vi "Loop_SEN.vi"() -> ()   [LabVIEW 2017, in "Dashboard.lvlib"]
uses:
  Dashboard.lvlib
  Globals/Global_STOP.vi
  Compressor/Globals/GLOBAL_ACT Write_Data_Out.vi
  Globals/Global_CMD_Drive.vi
  System_Monitoring/Global_SEN Write_Data.vi
  Globals/Global_CMD_Gear.vi
  Compressor/Compressor.lvlib
  System_Monitoring/System_Status.lvlib
panel:
  out "Cycle Time (S)":dbl format="%.3g"
  in  "Target Time(ms)":u32=50
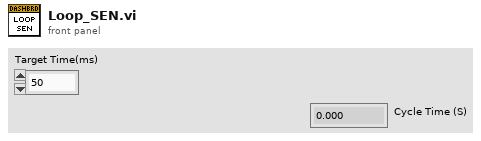
[diagram p1: front panel]
types:
  T1 = cluster{"Target Time(ms)":u32, "Current Time":timestamp, "Previous Time":timestamp, "Cycle Time (S)":dbl, "Num NET Vars":i32}
  T2 = typedef "Cluster_Compressor.ctl" = cluster{"Compressor Running":bool, "Compressor Enabled":bool}
  T3 = typedef "CLUSTER_CMD_WC_Drive.ctl" = cluster{"Drive_Mode":T4, "VBus":T5, "Profile":T7}
  T4 = typedef "ENUM_WC_Drive_DriveMode.ctl" = enum16{"Motion Profile", "CrossLineAuto", "VBus", "Stop"}
  T5 = typedef "CLUSTER_Drive_ACT Loop_VBus Data.ctl" = cluster{"Drive":T6, "Turbo":bool}
  T6 = typedef "CLUSTER_X and Y.ctl" = cluster{"Steer":dbl, "Throtle":dbl}
  T7 = typedef "CLUSTER_Drive_ACT Loop_Profile Data.ctl" = cluster{"Start":bool}
  T8 = typedef "CLUSTER_RoboRio_Status.ctl" = cluster{"RoboRio Faults":T9, "RIO inpt vol (V)":dbl, "RIO inpt cur (A)":dbl, "RoboRio Rails":T10}
  T9 = typedef "CLUSTER_RoboRio_Faults.ctl" = cluster{"Inpt. V. Brn. Out":bool, "3.3V Usr Rail Shrt.":bool, "5 V Usr Rail Shrt.":bool, "6 V Usr. Rail Shrt.":bool, "5V Usr. Rail Brn. Out":bool}
  T10 = typedef "CLUSTER_RoboRio_Rails.ctl" = cluster{"3.3 Volt":T11, "5 Volt":T11, "6 Volt":T11}
  T11 = typedef "CLUSTER_RoboRio_SingleRail.ctl" = cluster{"Vol.  (V)":dbl, "Cur. (A)":dbl}
  T12 = typedef "CLUSTER_PCM_Status.ctl" = cluster{"Current (A)":dbl, "All Solenoid Faults":bool[], "Input Voltage":dbl, "Solenoid Voltage":dbl, "Comp. Fault":bool}
  T13 = typedef "CLUSTER_PDP_Status.ctl" = cluster{"PDP Faults":T14, "All Currents (A)":dbl[], "Energy (J)":dbl, "Power (W)":dbl, "Voltage (V)":dbl}
  T14 = typedef "CLUSTER_PDP_Faults.ctl" = cluster{"Current Faults":bool[], "Batt V Fault":bool, "Temp Fault":bool, "HW Fault":bool}
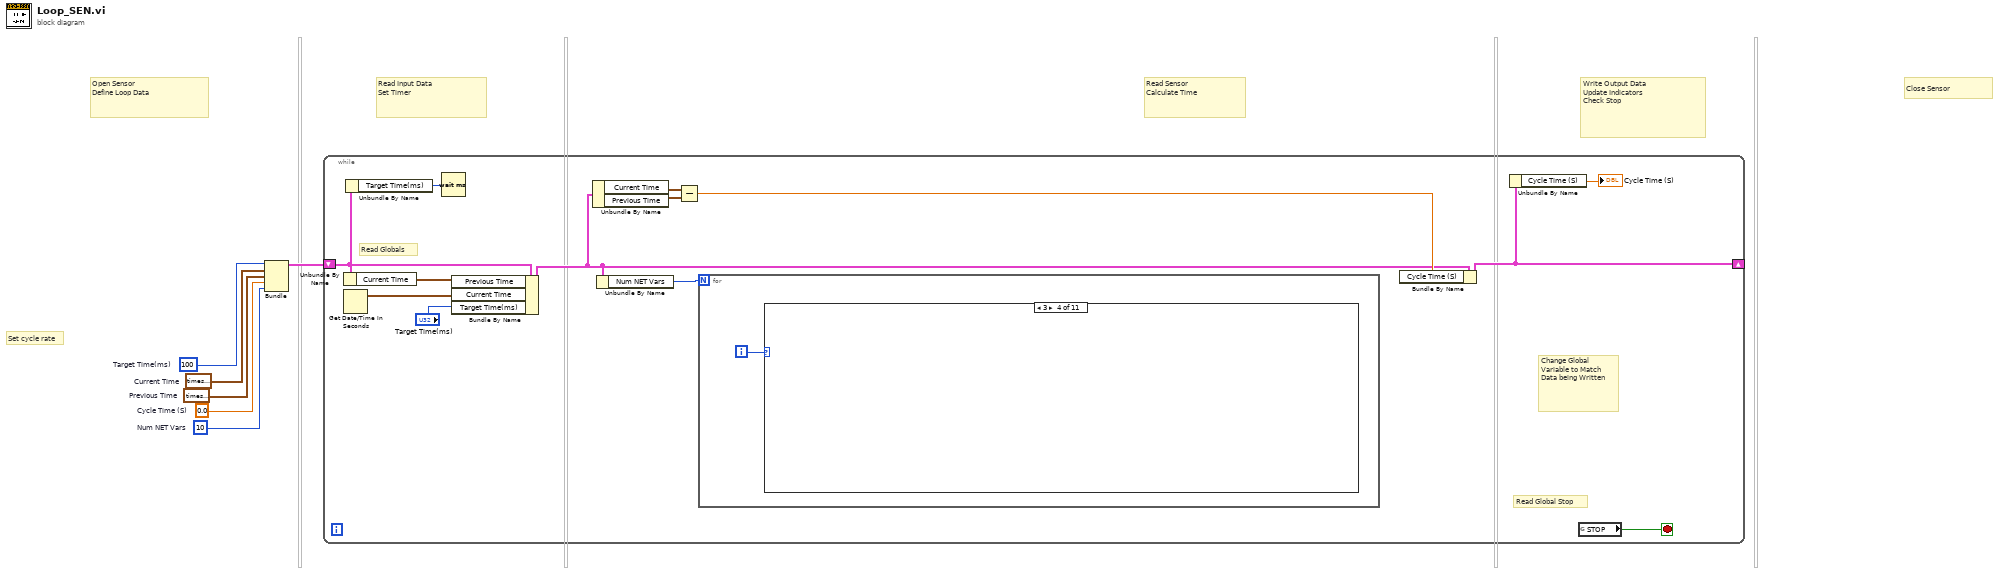
[diagram p0: block diagram]
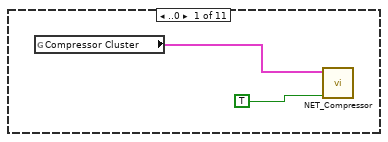
[diagram p2: hidden frame]
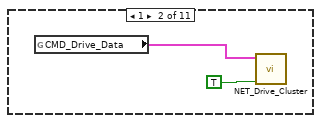
[diagram p3: hidden frame]
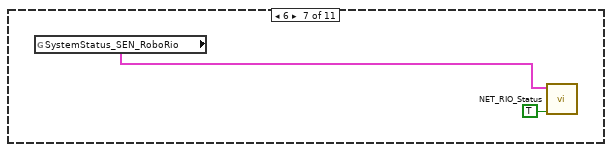
[diagram p7: hidden frame]
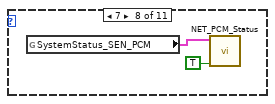
[diagram p8: hidden frame]
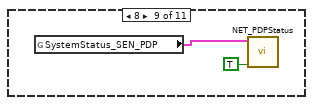
[diagram p9: hidden frame]
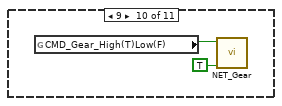
[diagram p10: hidden frame]
diagram:
  w1 = 10  # Num NET Vars
  w2 = 0.0  # Cycle Time (S)
  w6 = timestamp(0 s since 1904-01-01)  # Previous Time
  w5 = timestamp(0 s since 1904-01-01)  # Current Time
  w4 = u32 100  # Target Time(ms)
  # "Close Sensor"
  # "Write Output Data\nUpdate Indicators\nCheck Stop"
  # "Read Sensor\nCalculate Time"
  # "Read Input Data\nSet Timer"
  # "Open Sensor\nDefine Loop Data"
  # "Set cycle rate"
  n1 = Bundle("Target Time(ms)"=w4, "Current Time"=w5, "Previous Time"=w6, "Cycle Time (S)"=w2, "Num NET Vars"=w1) -> (w3:T1)  [unwired: 1 in]
  n2 = while {
    shift-right: [w11] -> _
    shift-left: w3 -> [w13]
    stop <- w19 stop-if-true
    # "Change Global\nVariable to Match\nData being Written"
    # "Read Globals"
    # "Read Global Stop"
    n3 = Unbundle By Name(w13) -> ("Current Time"=w17:timestamp)
    n4 = Get Date/Time In Seconds() -> (seconds since 1Jan1904=w18:timestamp)
    n5 = Unbundle By Name(w13) -> ("Target Time(ms)"=w12:u32)
    n6 = Wait (ms)(milliseconds to wait=w12) -> ()  [unwired: 1 out]
    n7 = Bundle By Name(cluster=w13, "Previous Time"=w17, "Current Time"=w18, "Target Time(ms)"="Target Time(ms)") -> (w8:T1)
    n8 = Unbundle By Name(w8) -> ("Current Time"=w16:timestamp, "Previous Time"=w15:timestamp)
    n9 = Unbundle By Name(w8) -> ("Num NET Vars"=w7:i32)
    n10 = Subtract(x=w16, y=w15) -> (x-y=w9:dbl)
    n11 = for {
      N: w7 -> [_]
      i -> [w20]
      n12 = case shown="3" w20 {
        frame ..0 {
          n13 = global read "GLOBAL_ACT Write_Data_Out.vi" "Compressor Cluster"() -> (w21:T2)
          n14 = call "NET_Compressor.vi"("Read(F) Write(T)"=TRUE, "Compressor  In"=w21) -> ()  [unwired: 9 in, 1 out]
        }
        frame 1 {
          n15 = global read "Global_CMD_Drive.vi" "CMD_Drive_Data"() -> (w23:T3)
          n16 = call "NET_Drive_Cluster.vi"("Read(F) Write(T)"=TRUE, "CMD_DriveCluster"=w23) -> ()  [unwired: 9 in, 1 out]
        }
        frame 2 {
        }
        frame 3 {
        }
        frame 4 {
        }
        frame 5 {
        }
        frame 6 {
          n17 = global read "Global_SEN Write_Data.vi" "SystemStatus_SEN_RoboRio"() -> (w25:T8)
          n18 = call "NET_RIO_Status.vi"("Read(F) Write(T)"=TRUE, "RoboRio Status In"=w25) -> ()  [unwired: 9 in, 1 out]
        }
        frame 7 {
          n19 = global read "Global_SEN Write_Data.vi" "SystemStatus_SEN_PCM"() -> (w28:T12)
          n20 = call "NET_PCM_Status.vi"("Read(F) Write(T)"=TRUE, "PCM_Status_In"=w28) -> ()  [unwired: 9 in, 1 out]
        }
        frame 8 {
          n21 = global read "Global_SEN Write_Data.vi" "SystemStatus_SEN_PDP"() -> (w30:T13)
          n22 = call "NET_PDPStatus.vi"("Read(F) Write(T)"=TRUE, "PDP_Status_In"=w30) -> ()  [unwired: 9 in, 1 out]
        }
        frame 9 {
          n23 = global read "Global_CMD_Gear.vi" "CMD_Gear_High(T)Low(F)"() -> (w31:bool)
          n24 = call "NET_Gear.vi"("Read(F) Write(T)"=TRUE, "High Gear In"=w31) -> ()  [unwired: 9 in, 1 out]
        }
        frame 10.. {
        }
      }
    }
    n25 = Bundle By Name(cluster=w8, "Cycle Time (S)"=w9) -> (w11:T1)
    n26 = Unbundle By Name(w11) -> ("Cycle Time (S)"=→"Cycle Time (S)":dbl)
    n27 = global read "Global_STOP.vi" "STOP"() -> (w19:bool)
  }
